vi "Meas.vi"(8 "error in (no error)":errorcluster, 10 "Wire in":T1, 11 "Gate in":refnum<class "G-UE.lvclass">) -> (0 "error out":errorcluster, 2 "Classical bit":bool, 3 "Gate out":refnum<class "G-UE.lvclass">)   [LabVIEW 2016, in "G-UE.lvclass"]
uses:
  G-UE.lvclass
  TypeDefs/Circuit Cluster.ctl
  GateAbst/GateAbst.lvclass
  G-UE.lvclass/G-UE.ctl
  <vilib>/Analysis/baseanly.llb/Complex A x Vector.vi
  <vilib>/Analysis/NI_AALBase.lvlib
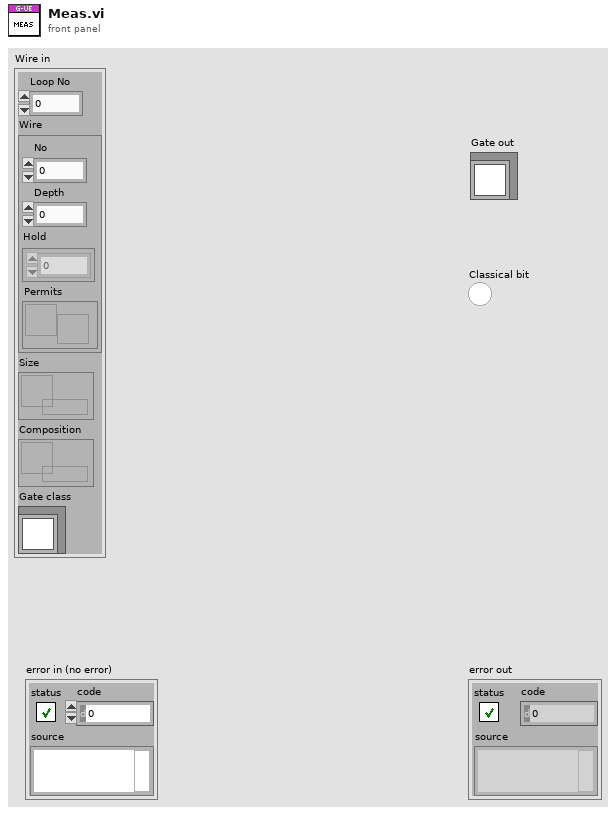
[diagram p1: front panel]
types:
  T1 = typedef "Circuit Cluster.ctl" = cluster{"Loop No":i32, "Wire":cluster{"No":i32, "Depth":i32, "Hold":i32[][], "Permits":refnum<notifier>}, "Size":refnum<queue>, "Composition":refnum<queue>, "Gate class":refnum<class "GateAbst.lvclass">}
  T2 = typedef "NI_Matrix.lvlib/ComplexMatrix.ctl" = cdb[][]
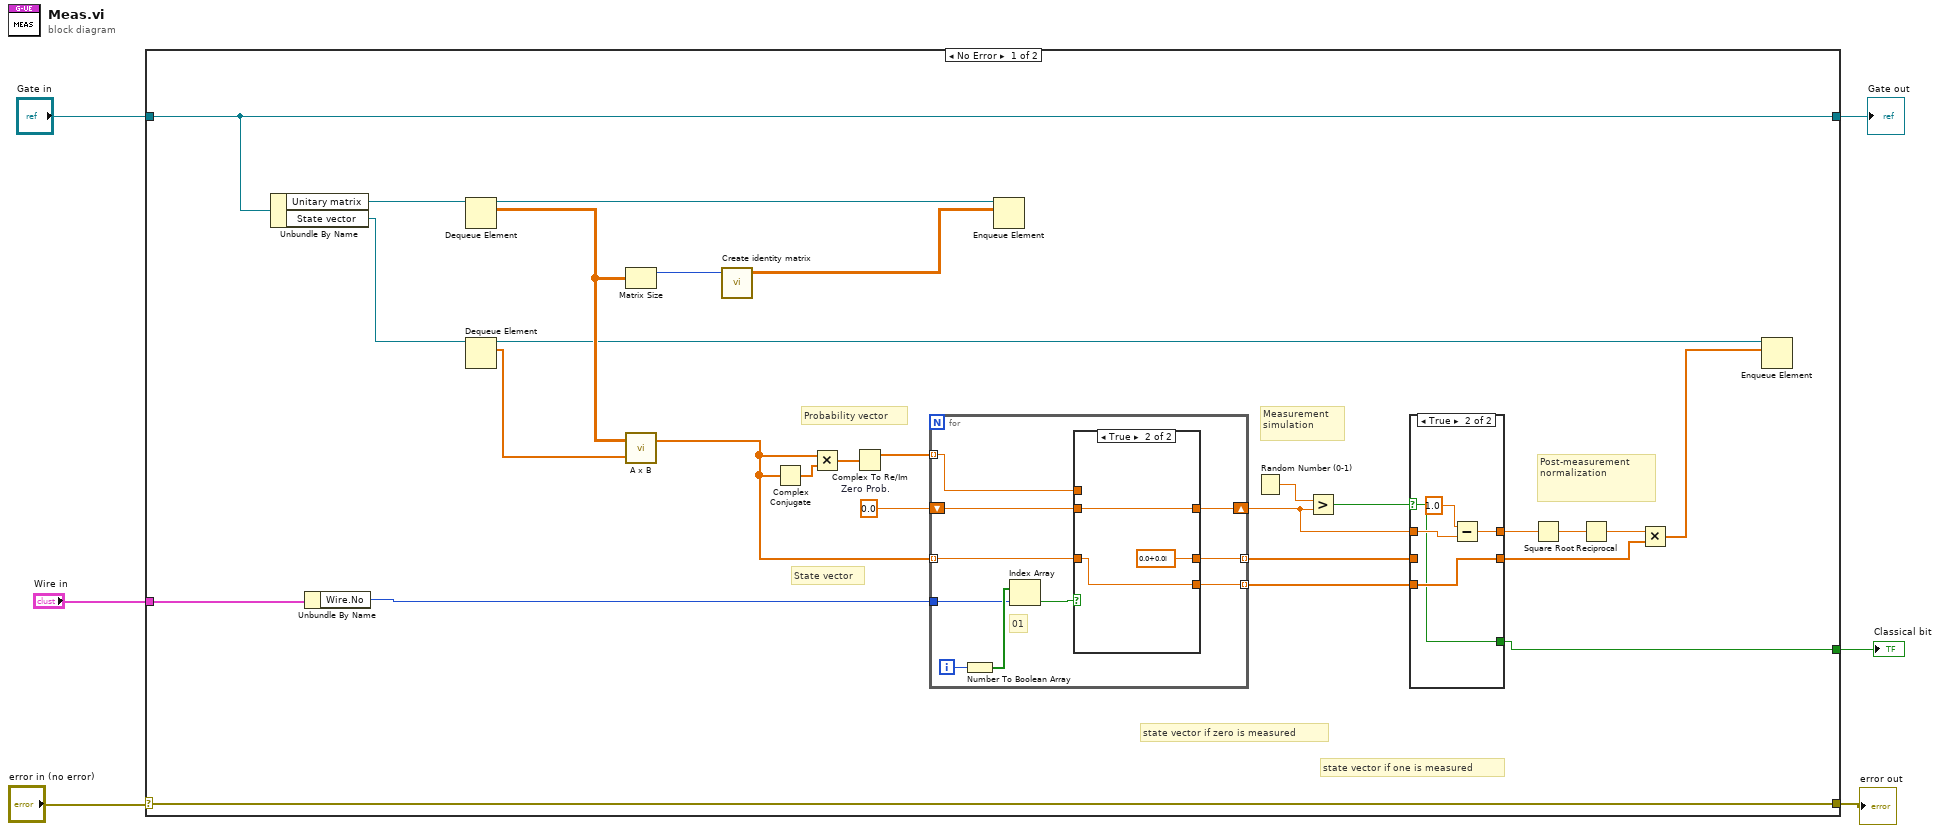
[diagram p0: block diagram]
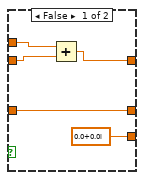
[diagram p2: hidden frame]
diagram:
  n1 = case shown="No Error" "error in (no error)" {
    selector: "error in (no error)" -> [w34 w62]
    tunnel: [w34 w62] -> w5
    tunnel: [w13 w61] -> w3
    tunnel: "Gate in" -> [w13 w61]
    tunnel: "Wire in" -> [w8 _]
    tunnel: [w7 _] -> w1
    frame No Error {
      w16 = 0.0  # Zero Prob.
      # "state vector if one is measured"
      # "state vector if zero is measured"
      # "State vector"
      # "Probability vector"
      # "Measurement\nsimulation"
      # "Post-measurement normalization"
      n2 = Unbundle By Name(w13) -> ("Unitary matrix"=w12:refnum<queue>, "State vector"=w10:refnum<queue>)
      n3 = Unbundle By Name(w8) -> ("Wire.No"=w15:i32)
      n4 = Dequeue Element(queue=w12) -> (queue out=w27:refnum<queue>, element=w28:T2)  [unwired: 2 in, 2 out]
      n5 = Dequeue Element(queue=w10) -> (queue out=w17:refnum<queue>, element=w33:cdb[])  [unwired: 2 in, 2 out]
      n6 = Matrix Size(0:w28) -> (1:w29:i32)  [unwired: 1 out]
      n7 = call-poly <vilib>:"A x B.vi"("Vector"=w33, "A"=w28) -> ("A x Vector"=w11:cdb[])  [unwired: 1 out]
      n8 = call "Create identity matrix.vi"("Matrix size"=w29) -> ("Identity Matrix"=w30:T2)  [unwired: 4 in]
      n9 = Complex Conjugate(1:w11) -> (0:w32:cdb[])
      n10 = Multiply ("Multiply.vi")(x=w11, y=w32) -> (x*y=w31:cdb[])
      n11 = Complex To Re/Im ("Complex To Cartesian.vi")(x + iy=w31) -> (x=w14:dbl[])  [unwired: 1 out]
      n12 = for {
        tunnel: w14 -> [w39] mode=indexing
        tunnel: w15 -> [w42]
        shift-right: [w38] -> w20
        shift-left: w16 -> [w40]
        tunnel: w11 -> [w37] mode=indexing
        tunnel: [w36] -> w21 mode=indexing
        tunnel: [w35] -> w22 mode=indexing
        i -> [w44]
        # "01"
        n13 = Number To Boolean Array(number=w44) -> (Boolean array=w43:bool[])
        n14 = Index Array "Index Array"(array=w43, index=w42) -> (element=w41:bool)
        n15 = case shown="True" w41 {
          tunnel: w40 -> [w49 w52]
          tunnel: w39 -> [w47 _]
          tunnel: [w48 w52] -> w38
          tunnel: w37 -> [w46 w51]
          tunnel: [w46 cdb 0.0+0.0i ("Complex Matrix Element")] -> w36
          tunnel: [cdb 0.0+0.0i ("Complex Matrix Element") w51] -> w35
          frame False {
            n16 = Add(x=w47, y=w49) -> (x+y=w48:dbl)
          }
          frame True {
          }
        }
      }
      n17 = Enqueue Element(queue=w27, element=w30) -> ()  [unwired: 2 in, 3 out]
      n18 = Random Number (0-1)() -> (number: 0 to 1=w18:dbl)
      n19 = Greater?(x=w18, y=w20) -> (0:w19:bool)
      n20 = case shown="True" w19 {
        selector: w19 -> [w53 w56]
        tunnel: w20 -> [w55 w60]
        tunnel: w21 -> [w54 _]
        tunnel: w22 -> [_ w57]
        tunnel: [w55 w58] -> w25
        tunnel: [w54 w57] -> w26
        tunnel: [w53 w56] -> w7
        frame False {
        }
        frame True {
          n21 = Subtract(x=1.0, y=w60) -> (x-y=w58:dbl)
        }
      }
      n22 = Square Root(x=w25) -> (sqrt(x)=w23:dbl)
      n23 = Reciprocal(x=w23) -> (1/x=w24:dbl)
      n24 = Multiply(x=w24, y=w26) -> (x*y=w9:cdb[])
      n25 = Enqueue Element(queue=w17, element=w9) -> ()  [unwired: 2 in, 3 out]
    }
    frame Error {
    }
  }
  "error out" <- w5
  "Gate out" <- w3
  "Classical bit" <- w1
